vi "帧12打包.vi"(0 "帧ID":i8 format="%x", 2 "D 6":i16, 3 "P1":i16, 4 "I 5":i16, 5 "P 4":i16, 6 "D 3":i16, 7 "I 2":i16) -> (1 "打包":string)   [LabVIEW 2016]
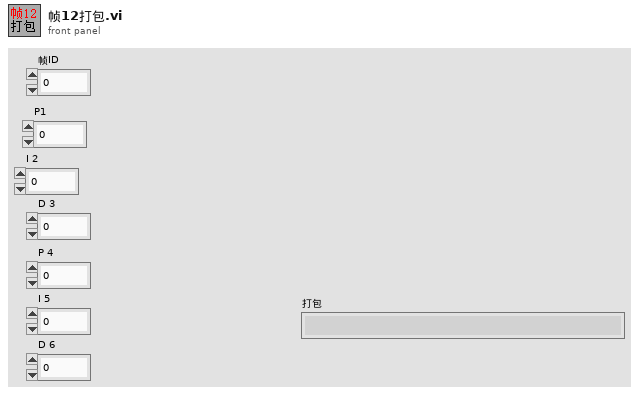
[diagram p1: front panel]
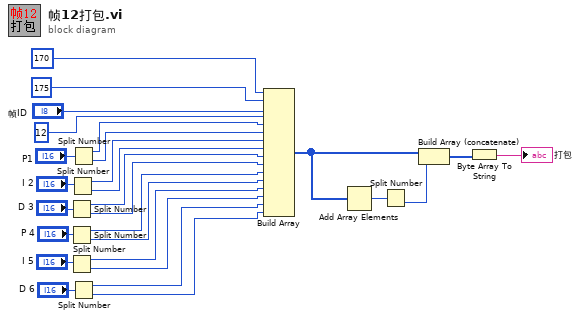
[diagram p0: block diagram]
diagram:
  n1 = Split Number(x="D 3") -> (hi(x)=w10:u8, lo(x)=w9:u8)
  n2 = Split Number(x="P 4") -> (hi(x)=w8:u8, lo(x)=w7:u8)
  n3 = Split Number(x="I 5") -> (hi(x)=w6:u8, lo(x)=w5:u8)
  n4 = Split Number(x="I 2") -> (hi(x)=w12:u8, lo(x)=w11:u8)
  n5 = Split Number(x="P1") -> (hi(x)=w14:u8, lo(x)=w13:u8)
  n6 = Split Number(x="D 6") -> (hi(x)=w4:u8, lo(x)=w3:u8)
  n7 = Build Array(170, 175, "帧ID", i8 12, w14, w13, w12, w11, w10, w9, w8, w7, w6, w5, w4, w3) -> (w26:i32[])
  n8 = Add Array Elements(numeric array=w26) -> (sum=w27:i32)
  n9 = Split Number(x=w27) -> (lo(x)=w1:u16)  [unwired: 1 out]
  n10 = Build Array (concatenate)(w26, w1) -> (w25:i32[])
  n11 = Byte Array To String(unsigned byte array=w25) -> (string=→"打包":string)
